vi "SV Convert Spectrum to Data Object.vi"(0 "spectrum":cluster{"f0":dbl, "df":dbl, "magnitude":dbl[]} {"magnitude" format="%.2p"; "df" format="%.2p"; "f0" format="%.2p"}, 4 "spectrum info":T1={"channel name"="", "description"="", "x-axis units"=0, "spectral info"={"spectrum type"=enum."Power [Magnitude^2]", "linear/dB"=enum."linear", "window"=0, "window size"=0, "FFT size"=0}, "engineering units"=0, "custom label"="", "dB reference [EU]"=0.0, "peak units"=enum."rms", "weighting filter"=0, "spectral density?"=FALSE, "unit label"="", "spectrum skewed?"=FALSE, "complimentary spectrum units"=enum."none"} {"x-axis units" items=["Time (s)"=0, "Frequency-CB (Hz)"=1, "Frequency-CPB (Hz)"=1248, "Frequency-Arbitrary (Hz)"=2357, "Quefrency (s)"=2, "Revolutions (rev)"=3, "Order"=4, "Speed (RPM)"=11, "Speed (rad/s)"=21, "Index"=65535]; "weighting filter" items=["Linear", "A-weighting", "B-weighting", "C-weighting", "ITU-R 468-4", "Dolby", "CCITT", "C-message", "Wb", "Wc", "Wd", "We", "Wf", "Wh", "Wj", "Wk", "Wm", "AES17 20 kHz lowpass", "AES17 40 kHz lowpass", "AES17 20 kHz highpass", "AES17 40 kHz highpass"]; "dB reference [EU]" format="%.2f"; "engineering units" items=["custom..."=0, "V"=1, "A"=21, "C"=30, "pC"=31, "s"=32, "-"=29, "Pa"=2, "N"=20, "g"=3, "m/s^2"=4, "m/s"=5, "m"=6, "mm/s"=12, "mm"=13, "micron/s"=14, "micron"=15, "in/s^2"=7, "in/s"=8, "in"=9, "mil/s"=10, "mil"=11, "rad/s^2"=16, "rad/s"=17, "rad"=18, "deg/s^2"=26, "deg/s"=27, "deg"=28, "RPM"=22, "cycle/s^2"=23, "Hz"=24, "cycle"=25, "strain"=19]; "spectral info"."window" items=["None "=0, "Hanning"=1, "Hamming"=2, "Blackman-Harris"=3, "Exact Blackman"=4, "Blackman"=5, "Flat Top"=6, "4 Term B-Harris "=7, "7 Term B-Harris"=8, "Low Sidelobe"=9, "Force - Exponential"=10, "Gaussian"=62]}, 5 "error in (no error)":errorcluster) -> (14 "Spectrum Data":refnum<class "Data.lvclass">, 19 "error out":errorcluster)   [LabVIEW 2017, in "Y (1 Ch).lvclass"]
doc: "Use this polymorphic VI to convert spectra to a class data type that you can view on the Spectrum with Cursors XControl. You must manually select the polymorphic instance to use."
uses:
  <vilib>/addons/_NISVFA/_Shared subVIs/Data Objects/Y (DBL)/Y (1 Ch).lvclass
  <vilib>/addons/_NISVFA/_Shared subVIs/Controls/svc_Spectrum Info.ctl
  <vilib>/addons/_NISVFA/_Shared subVIs/Controls/svc_X-Axis Units.ctl
  <vilib>/addons/_NISVFA/_Shared subVIs/Controls/svc_Spectrum Type.ctl
  <vilib>/addons/_NISVFA/_Shared subVIs/Controls/svc_Engineering Units Text Ring.ctl
  <vilib>/addons/_NISVFA/_Shared subVIs/Controls/svc_Weighting Filter Text Ring.ctl
  <vilib>/addons/_NISVFA/_Shared subVIs/Controls/svc_Complimentary Spectrum Units.ctl
  <vilib>/addons/_NISVFA/_Shared subVIs/Data Objects/Data/Data.lvclass
  C:/Program Files (x86)/National Instruments/LabVIEW 2017/vi.lib/addons/_NISVFA/_Shared subVIs/Data Objects/Data/Data.lvclass
  <vilib>/addons/_NISVFA/_Shared subVIs/Controls/NI Channel Properties.ctl
  <vilib>/addons/_NISVFA/_Shared subVIs/Data Objects/Data/Data.lvclass/Data.ctl
  <vilib>/addons/_NISVFA/_Shared subVIs/Data Objects/Data/Read Data Attributes.vi
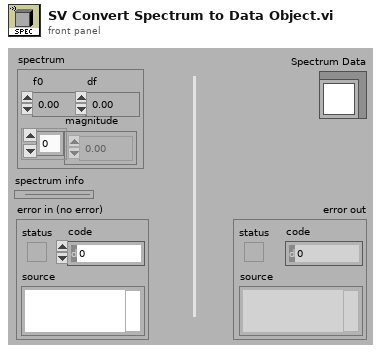
[diagram p1: front panel]
types:
  T1 = typedef "svc_Spectrum Info.ctl" = cluster{"channel name":string, "description":string, "x-axis units":T2, "spectral info":cluster{"spectrum type":T3, "linear/dB":enum16{"linear", "dB"}, "window":u16, "window size":i32, "FFT size":i32}, "engineering units":T4, "custom label":string, "dB reference [EU]":dbl, "peak units":enum16{"rms", "peak", "peak-peak"}, "weighting filter":T5, "spectral density?":bool, "unit label":string, "spectrum skewed?":bool, "complimentary spectrum units":T6}
  T2 = typedef "svc_X-Axis Units.ctl" = u16
  T3 = typedef "svc_Spectrum Type.ctl" = enum16{"FFT Spectrum [complex]", "Amplitude [Magnitude]", "Power [Magnitude^2]", "Cross Spectrum [complex]", "Frequency Response [Complex]"}
  T4 = typedef "svc_Engineering Units Text Ring.ctl" = u16
  T5 = typedef "svc_Weighting Filter Text Ring.ctl" = u16
  T6 = typedef "svc_Complimentary Spectrum Units.ctl" = enum16{"none", "radians", "degrees", "cycles", "imaginary"}
  T7 = typedef "NI Channel Properties.ctl" = u16
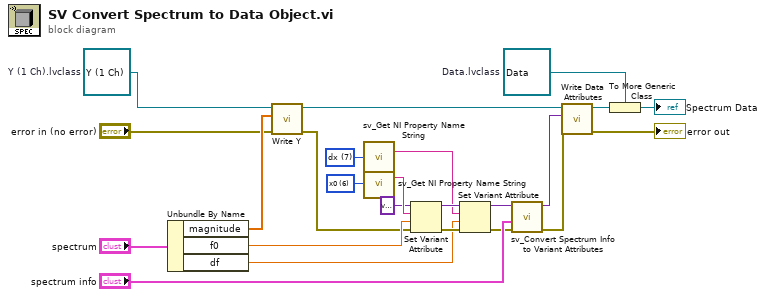
[diagram p0: block diagram]
diagram:
  w8 = refnum<class "Data.lvclass"> refnum  # Data.lvclass
  w14 = T7 6 items=["Channel name", "Channel description", "Axis label", "Unit string", "Waveform X-axis label", "Waveform X-axis unit string", "x0", "dx", "Number of samples", "X channel", "Filter settled", "dB reference", "Window", "Window parameter", "Window size", "FFT size", "Peak units", "Spectrum type", "Magnitude scale", "Spectral density", "Sensor sensitivity (mV/EU)", "X-axis dimension", "LabVIEW datatype", "Function type", "Function subtype", "X values", "Independent channel", "Column index", "Collection name", "Collection ID", "X Columns", "Phase unwrapped"] ("property")
  w15 = T7 7 items=["Channel name", "Channel description", "Axis label", "Unit string", "Waveform X-axis label", "Waveform X-axis unit string", "x0", "dx", "Number of samples", "X channel", "Filter settled", "dB reference", "Window", "Window parameter", "Window size", "FFT size", "Peak units", "Spectrum type", "Magnitude scale", "Spectral density", "Sensor sensitivity (mV/EU)", "X-axis dimension", "LabVIEW datatype", "Function type", "Function subtype", "X values", "Independent channel", "Column index", "Collection name", "Collection ID", "X Columns", "Phase unwrapped"] ("property")
  w11 = refnum<class "Y (1 Ch).lvclass"> refnum  # Y (1 Ch).lvclass
  n1 = Unbundle By Name("spectrum") -> ("magnitude"=w22:dbl[], "f0"=w17:dbl, "df"=w16:dbl)
  n2 = call <vilib>:"Write Y.vi"("error in (no error)"="error in (no error)", "Y"=w22, "Y (1Ch) in"=w11) -> ("error out"=w10:errorcluster, "Y (1Ch) out"=w5:refnum<class "Y (1 Ch).lvclass">)  [unwired: 7 in]
  n3 = call <vilib>:"sv_Get NI Property Name String.vi"("property"=w15) -> ("TDMS property name"=w12:string)  [unwired: 13 in, 1 out]
  n4 = call <vilib>:"sv_Get NI Property Name String.vi"("property"=w14) -> ("TDMS property name"=w13:string)  [unwired: 13 in, 1 out]
  n5 = Set Variant Attribute(Variant=variant ("data attributes"), name=w13, value=w17, error in=w10) -> (Variant out=w19:variant, error out=w20:errorcluster)  [unwired: 1 out]
  n6 = Set Variant Attribute(Variant=w19, name=w12, value=w16, error in=w20) -> (Variant out=w21:variant, error out=w18:errorcluster)  [unwired: 1 out]
  n7 = call <vilib>:"sv_Convert Spectrum Info to Variant Attributes.vi"("error in"=w18, "spectrum info"="spectrum info", "attributes in"=w21) -> ("error out"=w2:errorcluster, "attributes out"=w3:variant)  [unwired: 5 in, 2 out]
  n8 = call <vilib>:"Write Data Attributes.vi"("error in (no error)"=w2, "data attributes"=w3, "Data in"=w5) -> ("error out"=→"error out":errorcluster, "Data out"=w4:refnum<class "Y (1 Ch).lvclass">)  [unwired: 7 in]
  n9 = To More Generic Class(target class=w8, reference=w4) -> (generic class reference=→"Spectrum Data":refnum<class "Data.lvclass">)
